vi "E04_Tunel_SF.vi"() -> ()   [LabVIEW 2026]
panel:
  out "SF0 3":i32
  out "SF0 2":i32
  out "Arreglo (indexado)":i32[](array[numeric])
  out "SF0":i32
  out "Último valor":i32
  out "Shift register":i32
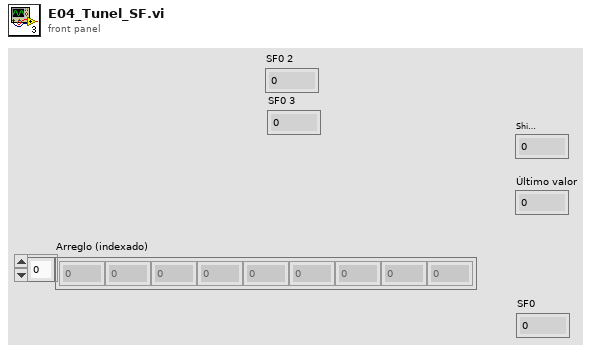
[diagram p1: front panel]
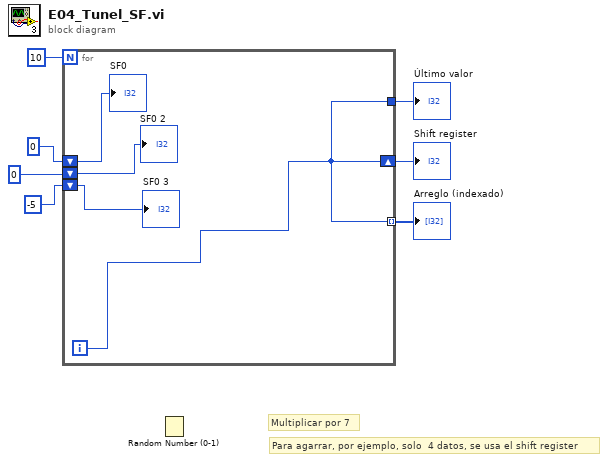
[diagram p0: block diagram]
diagram:
  # "Para agarrar, por ejemplo, solo  4 datos, se usa el shift register"
  # "Multiplicar por 7"
  n1 = for {
    N: 10 -> [_]
    shift-right: [w10] -> w6
    shift-left: 0 -> [w11]
    tunnel: [w10] -> w5
    tunnel: [w10] -> w4 mode=indexing
    shift-left: 0 -> [w8]
    shift-left: -5 -> [w9]
    i -> [w10]
    "SF0" <- w11
    "SF0 2" <- w8
    "SF0 3" <- w9
  }
  "Shift register" <- w6
  "Último valor" <- w5
  "Arreglo (indexado)" <- w4
  n2 = Random Number (0-1)() -> ()  [unwired: 1 out]
